vi "Apply Selected Labels to Control.vi"(8 "error in (no error)":errorcluster, 10 "Alternate Text Select (0)":i32, 11 "Table in":refnum<class "Table.lvclass">) -> (0 "error out":errorcluster, 3 "Table out":refnum<class "Table.lvclass">)   [LabVIEW 2017, in "Localization.lvlib" / "Table.lvclass"]
doc: "Use the information in the class to apply the selected alternate text from the Additional Labels to the control.\n\nChoose Movement Consulting, LLC"
uses:
  Table.lvclass
  C:/Apps/CMC/OpenSource/Localization/Control Info/Control Info.lvclass
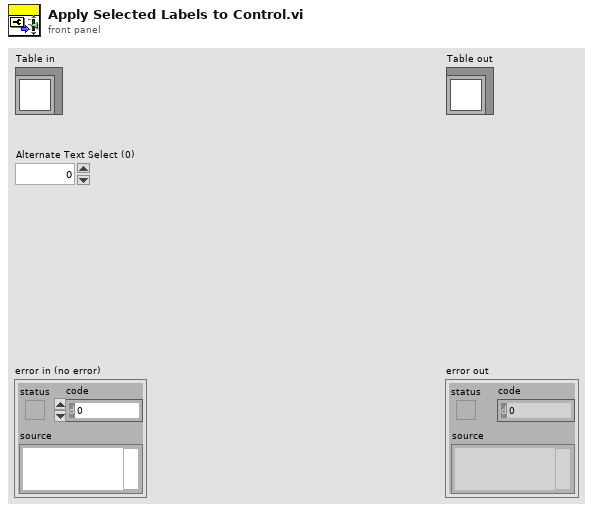
[diagram p1: front panel]
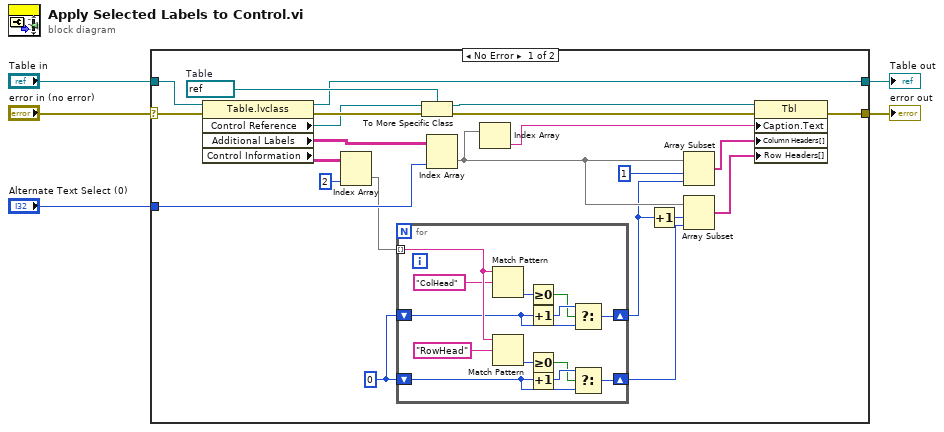
[diagram p0: block diagram]
diagram:
  n1 = case shown="No Error" "error in (no error)" {
    selector: "error in (no error)" -> [w23 w43]
    tunnel: "Table in" -> [w22 w42]
    tunnel: [w18 w43] -> w2
    tunnel: [w17 w42] -> w1
    tunnel: "Alternate Text Select (0)" -> [w20 _]
    frame No Error {
      w13 = 0
      w28 = refnum<vi> refnum  # Table
      n2 = property class="Table.lvclass"(reference=w22, error in=w23) -> (reference out=w17:refnum<class "Table.lvclass">, error out=w25:errorcluster, "Control Reference"=w24:refnum<vi>, "Additional Labels"=w21:string[][], "Control Information"=w16:string[][])
      n3 = Index Array(array=w16, index (col)=2 ("disabled index (col)")) -> (element=w14:string[])  [unwired: 1 in]
      n4 = for {
        tunnel: w14 -> [w41] mode=indexing
        shift-right: [w31] -> w9
        shift-left: w13 -> [w30]
        shift-right: [w35] -> w7
        shift-left: w13 -> [w34]
        n5 = Match Pattern(string=w41, regular expression="ColHead") -> (offset past match=w38:i32)  [unwired: 1 in, 3 out]
        n6 = Match Pattern(string=w41, regular expression="RowHead") -> (offset past match=w37:i32)  [unwired: 1 in, 3 out]
        n7 = Greater Or Equal To 0?(x=w38) -> (x >= 0?=w33:bool)
        n8 = Increment(x=w34) -> (x+1=w36:i32)
        n9 = Greater Or Equal To 0?(x=w37) -> (x >= 0?=w29:bool)
        n10 = Increment(x=w30) -> (x+1=w32:i32)
        n11 = Select(t=w36, s=w33, f=w34) -> (s? t:f=w35:i32)
        n12 = Select(t=w32, s=w29, f=w30) -> (s? t:f=w31:i32)
      }
      n13 = To More Specific Class(target class=w28, reference=w24, error in=w25) -> (specific class reference=w27:refnum<vi>, error out=w26:errorcluster)
      n14 = Index Array(array=w21, index (col)=w20) -> (element=w10:string[])  [unwired: 1 in]
      n15 = Index Array(array=w10) -> (element=w19:string)  [unwired: 1 in]
      n16 = Increment(x=w7) -> (x+1=w6:i32)
      n17 = Array Subset(array=w10, index=1, length=w7) -> (w11:string[])
      n18 = Array Subset(array=w10, index=w6, length=w9) -> (w8:string[])
      n19 = property class="Tbl"(reference=w27, error in=w26, "Caption.Text"=w19, "Column Headers[]"=w11, "Row Headers[]"=w8) -> (error out=w18:errorcluster)  [unwired: 1 out]
    }
    frame Error {
    }
  }
  "error out" <- w2
  "Table out" <- w1
